vi "PCO_Live.vi"(7 "Message Data":variant, 8 "entrée d'erreur (pas d'erreur)":errorcluster, 9 "notifier in":refnum<notifier>, 10 "dup Message Queue":refnum<queue>, 11 "Camera en entrée":refnum<class "Camera.lvclass">) -> (0 "sortie d'erreur":errorcluster, 3 "Camera en sortie":refnum<class "Camera.lvclass">)   [LabVIEW 2026]
uses:
  QMH/Message Queue/Message Cluster.ctl
  pco.labview/camera/Camera.lvclass
  Controls/PCO_Config.ctl
  Controls/TypeDef_FGV.ctl
  QMH/Message Queue/Message Queue.lvlib
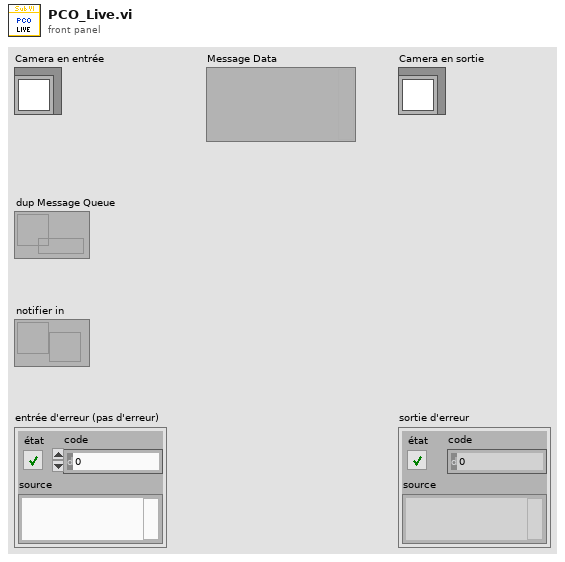
[diagram p1: front panel]
types:
  T1 = enum16{"sequence", "sequence non blocking", "ring buffer", "fifo", "tif", "multitif", "pcoraw", "b16", "dicom", "multidicom", "camram_ring", "camram_segment"}
  T2 = typedef "PCO_Config.ctl" = cluster{"Exposure time (s)":dbl, "TriggerMode":u16, "ROI X0":u16, "ROI Y0":u16, "ROI X1":u16, "ROI Y1":u16, "Binning":u8}
  T3 = typedef "TypeDef_FGV.ctl" = enum16{"Initialize", "Write", "Read"}
  T4 = enum16{"Undefined", "Mono8", "Mono16", "BGRA8", "RGBA8", "BGRA16", "RGBA16", "CompressedMono8"}
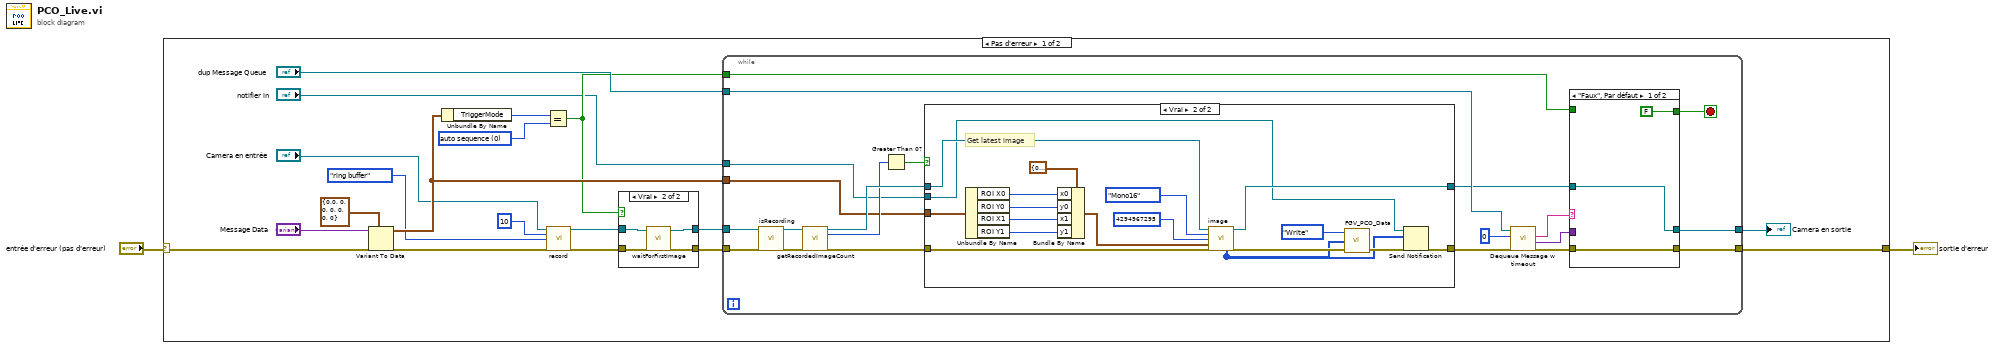
[diagram p0: block diagram]
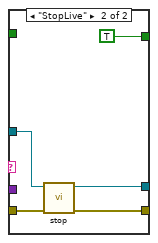
[diagram p2: hidden frame]
diagram:
  n1 = case shown="Pas d'erreur" "entrée d'erreur (pas d'erreur)" {
    selector: "entrée d'erreur (pas d'erreur)" -> [w6 w77]
    tunnel: [w17 w77] -> w2
    frame No Error {
      w11 = u16 0 items=["auto sequence", "software trigger", "external exposure start", "external exposure control"] ("TriggerMode")
      n2 = Variant To Data(error in=w6, type=T2 {"Exposure time (s)"=0.0, "TriggerMode"=0, "ROI X0"=0, "ROI Y0"=0, "ROI X1"=0, "ROI Y1"=0, "Binning"=0} ("PCO_Config"), Variant="Message Data") -> (data=w16:T2, error out=w10:errorcluster)
      n3 = Unbundle By Name(w16) -> ("TriggerMode"=w12:u16)
      n4 = Equal?(x=w12, y=w11) -> (x = y?=w5:bool)
      n5 = call-dynamic "record.vi"("Camera in"="Camera en entrée", "num_images"=u32 10 ("dwImgCount"), "record_mode"=T1."ring buffer", "error in (no error)"=w10) -> ("Camera out"=w20:refnum<class "Camera.lvclass">, "error out"=w19:errorcluster)  [unwired: 10 in]
      n6 = case shown="Vrai" w5 {
        tunnel: w19 -> [w71 w76]
        tunnel: w20 -> [w72 w75]
        tunnel: [w72 w74] -> w15
        tunnel: [w71 w73] -> w14
        frame False {
        }
        frame True {
          n7 = call-dynamic "waitForFirstImage.vi"("error in (no error)"=w76, "Camera in"=w75) -> ("error out"=w73:errorcluster, "Camera out"=w74:refnum<class "Camera.lvclass">)  [unwired: 8 in]
        }
      }
      n8 = while {
        tunnel: w14 -> [w36]
        tunnel: w15 -> [w35]
        tunnel: w16 -> [w34]
        tunnel: "dup Message Queue" -> [w32]
        tunnel: [w27] -> w17
        tunnel: [w26] -> w18
        tunnel: w5 -> [w23]
        tunnel: "notifier in" -> [w22]
        stop <- w25 stop-if-true
        n9 = call-dynamic "isRecording.vi"("Camera in"=w35, "error in (no error)"=w36) -> ("Camera out"=w42:refnum<class "Camera.lvclass">, "error out"=w41:errorcluster)  [unwired: 11 in, 1 out]
        n10 = call-dynamic "getRecordedImageCount.vi"("Camera in"=w42, "error in (no error)"=w41) -> ("Camera out"=w39:refnum<class "Camera.lvclass">, "recorded_image_count"=w37:u32, "error out"=w40:errorcluster)  [unwired: 11 in]
        n11 = Greater Than 0?(x=w37) -> (x > 0?=w38:bool)
        n12 = case shown="Vrai" w38 {
          tunnel: [w51 w55] -> w33
          tunnel: w40 -> [w51 w67]
          tunnel: w39 -> [w52 w66]
          tunnel: [w52 w65] -> w28
          tunnel: w34 -> [_ w64]
          tunnel: w22 -> [_ w54]
          frame False {
          }
          frame True {
            # "Get latest image"
            n13 = Unbundle By Name(w64) -> ("ROI X0"=w63:u16, "ROI Y0"=w62:u16, "ROI X1"=w61:u16, "ROI Y1"=w60:u16)
            n14 = Bundle By Name(cluster=cluster{"x0":u64, "y0":u64, "x1":u64, "y1":u64} {"x0"=0, "y0"=0, "x1"=0, "y1"=0} ("roi"), "x0"=w63, "y0"=w62, "x1"=w61, "y1"=w60) -> (w68:cluster{"x0":u64, "y0":u64, "x1":u64, "y1":u64})
            n15 = call-dynamic "image.vi"("Camera in"=w66, "data_format"=T4."Mono16", "image_index"=u32 4294967295 ("dwImgIdx"), "crop"=w68, "error in (no error)"=w67) -> ("Camera out"=w65:refnum<class "Camera.lvclass">, "raw_image (U16)"=w53:u16[][], "error out"=w57:errorcluster)  [unwired: 2 in, 6 out]
            n16 = call "FGV_PCO_Data.vi"("error in"=w57, "Data"=w53, "Action"=TypeDef_FGV."Write") -> ("error out"=w56:errorcluster)  [unwired: 1 in, 1 out]
            n17 = Send Notification(notification=w53, notifier=w54, error in (no error)=w56) -> (error out=w55:errorcluster)  [unwired: 1 out]
          }
        }
        n18 = call "Dequeue Message w timeout.vi"("entrée d'erreur (pas d'erreur)"=w33, "timeout en ms (-1)"=0, "Message Queue"=w32) -> ("sortie d'erreur"=w30:errorcluster, "Message Data"=w29:variant, "Message"=w31:string)  [unwired: 5 in, 1 out]
        n19 = case shown="\"Faux\", Par défaut" w31 {
          tunnel: w30 -> [w44 w49]
          tunnel: w29 -> [_ _]
          tunnel: w28 -> [w45 w50]
          tunnel: [w44 w48] -> w27
          tunnel: [w45 w47] -> w26
          tunnel: [FALSE TRUE] -> w25
          tunnel: w23 -> [_ _]
          frame "Faux", Default {
          }
          frame "StopLive" {
            n20 = call-dynamic "stop.vi"("error in (no error)"=w49, "Camera in"=w50) -> ("error out"=w48:errorcluster, "Camera out"=w47:refnum<class "Camera.lvclass">)  [unwired: 8 in]
          }
        }
      }
      "Camera en sortie" <- w18
    }
    frame Error {
    }
  }
  "sortie d'erreur" <- w2
